vi "Format Error.vi"(8 "error in (no error)":errorcluster, 9 "Additional source description":string, 10 "error message":string, 11 "error code":i32) -> (0 "error out":errorcluster)   [LabVIEW 2023, in "SQLiteSupport.lvlib"]
uses:
  SQLiteSupport.lvlib
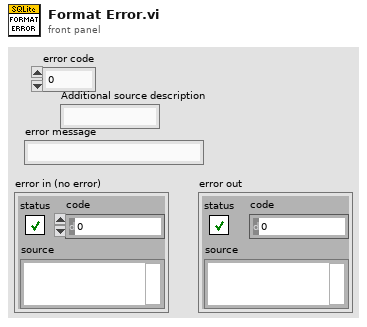
[diagram p1: front panel]
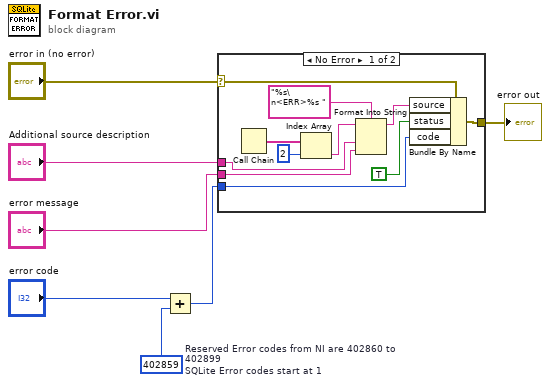
[diagram p0: block diagram]
diagram:
  w2 = 402859  # Reserved Error codes from NI are 402860 to 402899 SQLite Error codes start at 1
  n1 = Add(x="error code", y=w2) -> (x+y=w4:i32)
  n2 = case shown="No Error" "error in (no error)" {
    selector: "error in (no error)" -> [w14 w19]
    tunnel: "error message" -> [w16 _]
    tunnel: w4 -> [w13 _]
    tunnel: [w15 w19] -> w5
    tunnel: "Additional source description" -> [w8 _]
    frame No Error {
      n3 = Call Chain() -> (call chain=w11:string[])
      n4 = Index Array(array=w11, index=2) -> (element=w10:string)
      n5 = Format Into String(format string="%s\n<ERR>%s ", initial string=w10, w8, w16) -> (resulting string=w18:string)  [unwired: 1 in, 1 out]
      n6 = Bundle By Name(cluster=w14, "source"=w18, "status"=TRUE, "code"=w13) -> (w15:errorcluster)
    }
    frame Error {
    }
  }
  "error out" <- w5
